vi "VLC-IP_MediePlayer&Media_Initialize.vi"(8 "error in (no error)":errorcluster, 10 "Script":string, 11 "Media Source":string="rtsp://admin:admin@192.168.1.108/cam/realmonitor?channel=1&subtype=1") -> (0 "error out":errorcluster, 3 "VLC-IP":T1)   [LabVIEW 2016]
uses:
  VLC-IP.ctl
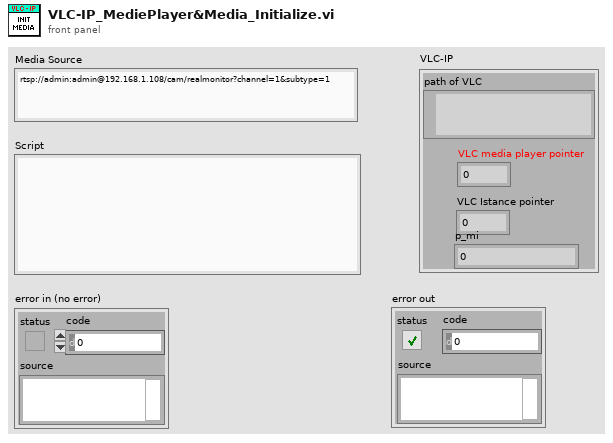
[diagram p1: front panel]
types:
  T1 = typedef "VLC-IP.ctl" = cluster{"path of VLC":path, "VLC media player pointer":i32, "VLC Istance pointer":i32, "p_mi":i32}
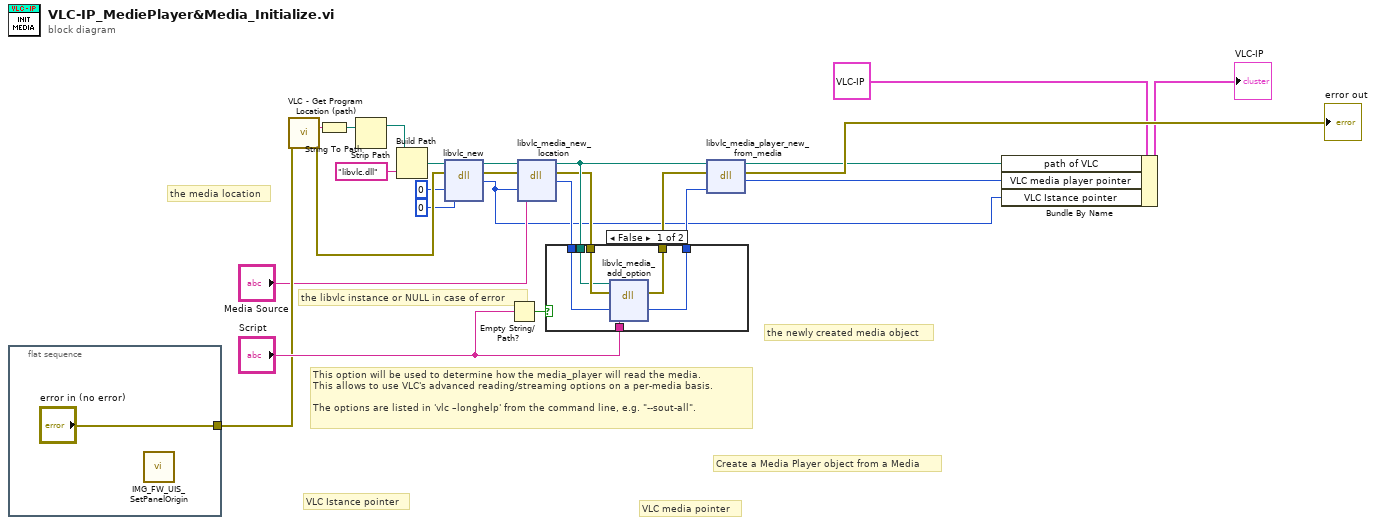
[diagram p0: block diagram]
diagram:
  # "VLC media pointer"
  # "VLC Istance pointer"
  # "Create a Media Player object from a Media"
  # "This option will be used to determine how the media_player will read the media. \nThis allows to use VLC's advanced reading/streaming options on a per-media basis.\n\nThe options are listed in 'vlc –longhelp' from the command line, e.g. \"--sout-all\"."
  # "the newly created media object"
  # "the media location"
  # "the libvlc instance or NULL in case of error"
  n1 = flat-sequence {
    tunnel: ["error in (no error)"] -> w20
    frame #0 {
      n2 = call "IMG_FW_UIS_SetPanelOrigin.vi"() -> ()  [unwired: 11 in, 1 out]
    }
  }
  n3 = call "VLC - Get Program Location (path).vi"("error in (no error)"=w20) -> ("VLC path"=w15:string, "error out"=w21:errorcluster)  [unwired: 13 in]
  n4 = String To Path(string=w15) -> (path=w16:path)
  n5 = Strip Path(path=w16) -> (stripped path=w25:path)  [unwired: 1 out]
  n6 = Build Path(base path=w25, name or relative path="libvlc.dll") -> (appended path=w18:path)
  n7 = dll-call lib="C:/Program Files (x86)/VideoLAN/VLC/libvlc.dll" fn="libvlc_new"(path in=w18, error in=w21, "argc"=i16 0, "argv"=u8 0) -> (path out=w14:path, error out=w11:errorcluster, "return type"=w1:i32)  [unwired: 3 in]
  n8 = Empty String/Path?(string/path="Script") -> (empty?=w23:bool)
  n9 = dll-call lib="C:/Program Files (x86)/VideoLAN/VLC/libvlc.dll" fn="libvlc_media_new_location"(path in=w14, error in=w11, "p_instance"=w1, "path"="Media Source") -> (path out=w24:path, error out=w9:errorcluster, "return type"=w8:i32)  [unwired: 3 in]
  n10 = case shown="False" w23 {
    tunnel: w9 -> [w32 w34]
    tunnel: w8 -> [w31 w33]
    tunnel: [w30 w33] -> w7
    tunnel: [w29 w34] -> w6
    tunnel: "Script" -> [w28 _]
    tunnel: w24 -> [w27 _]
    frame False {
      n11 = dll-call lib="C:/Program Files (x86)/VideoLAN/VLC/libvlc.dll" fn="libvlc_media_add_option"(path in=w27, error in=w32, "p_md"=w31, "ppsz_options"=w28) -> (error out=w29:errorcluster, "p_md"=w30:i32)  [unwired: 3 in, 1 out]
    }
    frame True {
    }
  }
  n12 = dll-call lib="C:/Program Files (x86)/VideoLAN/VLC/libvlc.dll" fn="libvlc_media_player_new_from_media"(path in=w24, error in=w6, "p_md"=w7) -> (path out=w3:path, error out=→"error out":errorcluster, "return type"=w2:i32)  [unwired: 2 in]
  n13 = Bundle By Name(cluster=T1 {"path of VLC"=path "C:/Program Files (x86)/VideoLAN/VLC/libvlc.dll", "VLC media player pointer"=858078584, "VLC Istance pointer"=862402584, "p_mi"=0} ("VLC-IP"), "path of VLC"=w3, "VLC media player pointer"=w2, "VLC Istance pointer"=w1) -> (→"VLC-IP":T1)
